vi "Get Broadcast Event Recursively.vi"(8 "error in (no error)":errorcluster, 11 "Application in":refnum<class "Application.lvclass">) -> (0 "error out":errorcluster, 2 "Broadcast Event":refnum<user-event>[](array[refnum]), 3 "Application out":refnum<class "Application.lvclass">)   [LabVIEW 2020, in "Application.lvclass"]
doc: "Get the broadcast event used to send broadcasts to registered observers."
uses:
  Application.lvclass
  C:/Users/anton/Documents/GitHub/Triarc-Framework/source/Framework/Process/Process.lvclass
  Process/Protected/Broadcasting/Broadcast Message Cluster.ctl
  Process/Process.lvclass/Process.ctl
  Application.lvclass/Application.ctl
  Process/Public/Lifecycle/Get Lifecycle State.vi
  Process/Protected/Messaging/Request Message.vi
  <vilib>/Utility/error.llb/Clear Errors.vi
  Process/Private/SubVIs/Enqueue Request Message.vi
  <vilib>/AdvancedString/1D String Array to Delimited String.vi
  <vilib>/Utility/error.llb/Error Cluster From Error Code.vi
  Process/Private/SubVIs/Wait for Response Message.vi
  Process/Process.lvclass
  C:/Users/anton/Documents/GitHub/Triarc-Framework/source/Framework/Base/Base.lvclass
  C:/Users/anton/Documents/GitHub/Triarc-Framework/source/Framework/Error Handler Interface/Error Handler Interface.lvclass
  C:/Users/anton/Documents/GitHub/Triarc-Framework/source/Framework/Application/Application.lvclass
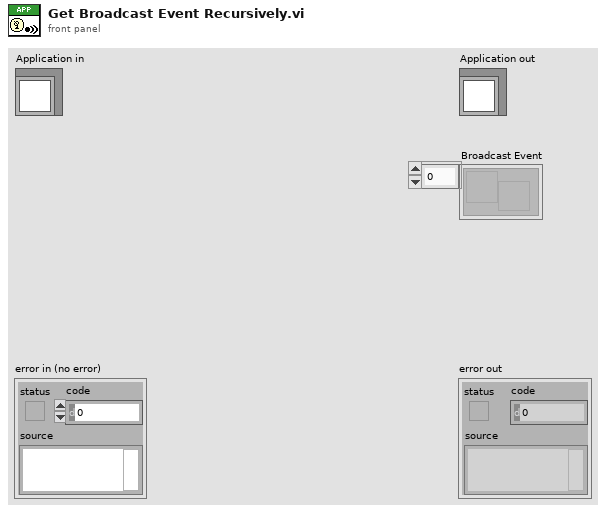
[diagram p1: front panel]
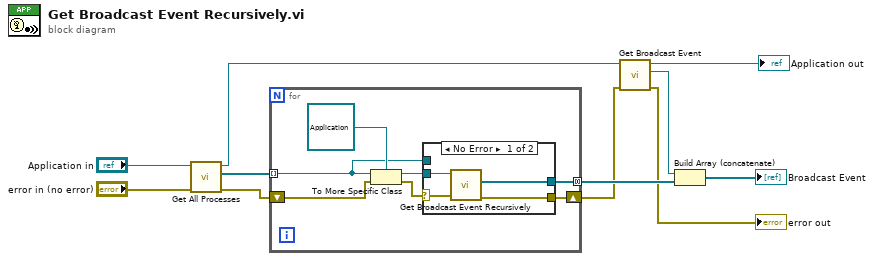
[diagram p0: block diagram]
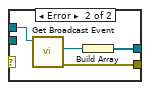
[diagram p2: hidden frame]
diagram:
  n1 = call "Get All Processes.vi"("error in (no error)"="error in (no error)", "Application In"="Application in") -> ("error out"=w9:errorcluster, "App Processes"=w11:refnum<class "Process.lvclass">[], "Application Out"=w7:refnum<class "Application.lvclass">)  [unwired: 7 in]
  n2 = for {
    tunnel: w11 -> [w12] mode=indexing
    tunnel: [w13] -> w10 mode=concatenating
    shift-right: [w14] -> w6
    shift-left: w9 -> [w17]
    n3 = To More Specific Class(target class=refnum<class "Application.lvclass"> refnum ("Application in"), reference=w12, error in=w17) -> (specific class reference=w16:refnum<class "Application.lvclass">, error out=w15:errorcluster)
    n4 = case shown="No Error" w15 {
      selector: w15 -> [w21 _]
      tunnel: w16 -> [w22 _]
      tunnel: [w20 w26] -> w14
      tunnel: [w19 w24] -> w13
      tunnel: w12 -> [_ w23]
      frame No Error {
        n5 = call-dynamic "Get Broadcast Event Recursively.vi"("error in (no error)"=w21, "Application in"=w22) -> ("error out"=w20:errorcluster, "Broadcast Event"=w19:refnum<user-event>[])  [unwired: 7 in, 1 out]
      }
      frame Error {
        n6 = call "Get Broadcast Event.vi"("Process in"=w23) -> ("error out"=w26:errorcluster, "Broadcast Event"=w25:refnum<user-event>)  [unwired: 8 in, 1 out]
        n7 = Build Array(w25) -> (w24:refnum<user-event>[])
      }
    }
  }
  n8 = call "Get Broadcast Event.vi"("error in (no error)"=w6, "Process in"=w7) -> ("error out"=→"error out":errorcluster, "Broadcast Event"=w8:refnum<user-event>, "Process out"=→"Application out":refnum<class "Application.lvclass">)  [unwired: 7 in]
  n9 = Build Array (concatenate)(w8, w10) -> (→"Broadcast Event":refnum<user-event>[])
